vi "avgSpectra.vi"() -> ()   [LabVIEW 2020]
uses:
  <vilib>/Utility/file.llb/Write Delimited Spreadsheet (DBL).vi
  <instrlib>/Ocean Optics 2000 4000/Ocean Optics 2000 4000.lvlib
panel:
  out "Array":dbl[](array[numeric])
  in  "Enable Strobe (Disabled)":bool
  out "Spectral Waveform":cluster{dbl[], dbl[]}(graph)
  in  "VISA resource name":refnum<visa-resource-name>
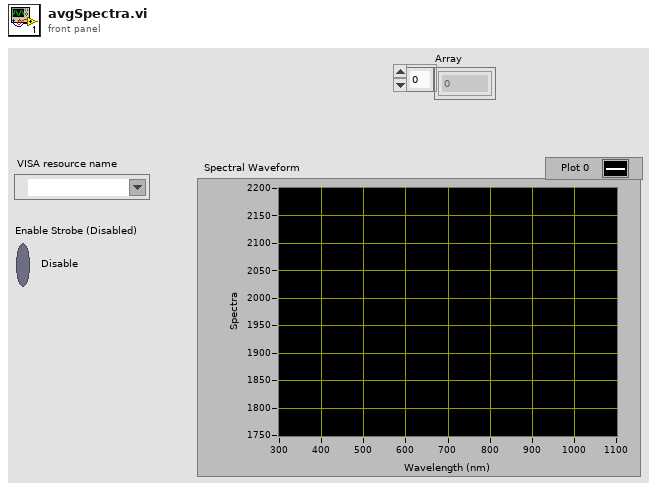
[diagram p1: front panel]
types:
  T1 = cluster{"Wavelength (nm)":dbl[], "Spectrum by Pixel Number":dbl[]}
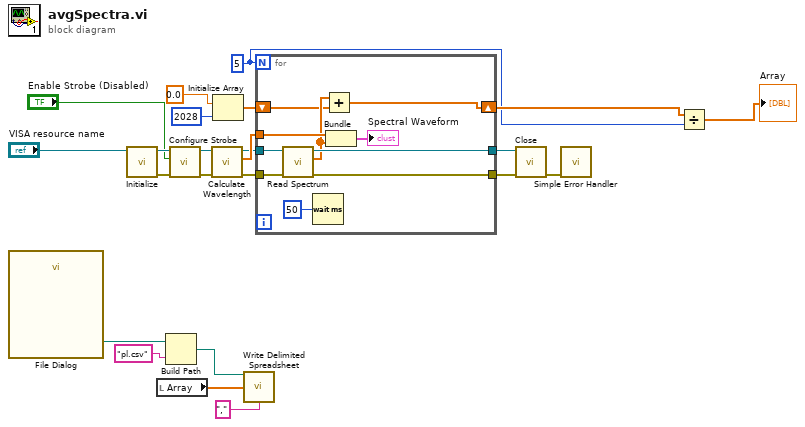
[diagram p0: block diagram]
diagram:
  w2 = 5
  n1 = call "File Dialog"() -> ("selected path"=w8:path)  [unwired: 12 in, 3 out]
  n2 = call <instrlib>:"Initialize.vi"("VISA resource name"="VISA resource name") -> ("error out"=w22:errorcluster, "VISA resource name out"=w23:refnum<visa-resource-name>)  [unwired: 2 in, 7 out]
  n3 = local read "Array"() -> (w4:dbl[])
  n4 = Build Path(base path=w8, name or relative path="pl.csv") -> (appended path=w5:path)
  n5 = call <instrlib>:"Configure Strobe.vi"("error in (no error)"=w22, "Enable Strobe (Disabled)"="Enable Strobe (Disabled)", "VISA resource name"=w23) -> ("error out"=w12:errorcluster, "VISA resource name out"=w13:refnum<visa-resource-name>)  [unwired: 7 out]
  n6 = call <instrlib>:"Calculate Wavelength.vi"("error in (no error)"=w12, "VISA resource name"=w13) -> ("error out"=w14:errorcluster, "Wavelength (nm)"=w16:dbl[], "VISA resource name out"=w15:refnum<visa-resource-name>)  [unwired: 1 in, 6 out]
  n7 = Initialize Array(0.0 ("element"), 2028 ("dimension size")) -> (w9:dbl[])
  n8 = call-poly <vilib>:"Write Delimited Spreadsheet.vi"("file path (dialog if empty)"=w5, "1D data"=w4, "delimiter (\\t)"=",") -> ()  [unwired: 11 in, 2 out]
  n9 = for {
    N: w2 -> [_]
    tunnel: [w32] -> w20
    tunnel: [w31] -> w19
    tunnel: w16 -> [w30]
    tunnel: w15 -> [w29]
    tunnel: w14 -> [w28]
    shift-right: [w24] -> w3
    shift-left: w9 -> [w25]
    n10 = call <instrlib>:"Read Spectrum.vi"("error in (no error)"=w28, "VISA resource name"=w29) -> ("error out"=w31:errorcluster, "Spectrum by Pixel Number"=w26:dbl[], "VISA resource name out"=w32:refnum<visa-resource-name>)  [unwired: 6 in, 1 out]
    n11 = Wait (ms)(milliseconds to wait=u32 50 ("millisecond multiple")) -> ()  [unwired: 1 out]
    n12 = Add(x=w26, y=w25) -> (x+y=w24:dbl[])
    n13 = Bundle("Wavelength (nm)"=w30, "Spectrum by Pixel Number"=w26) -> (→"Spectral Waveform":T1)  [unwired: 1 out]
  }
  n14 = call <instrlib>:"Close.vi"("error in (no error)"=w19, "VISA resource name"=w20) -> ("error out"=w18:errorcluster)  [unwired: 9 out]
  n15 = call <vilib>:"Simple Error Handler.vi"("error in (no error)"=w18) -> ()  [unwired: 1 in, 8 out]
  n16 = Divide(x=w3, y=w2) -> (x/y=→"Array":dbl[])
